vi "Display.vi"() -> ()   [LabVIEW 2009]
panel:
  out "waveform":cluster{i32, dbl, dbl[][]}(graph)
  # "Panel 1"
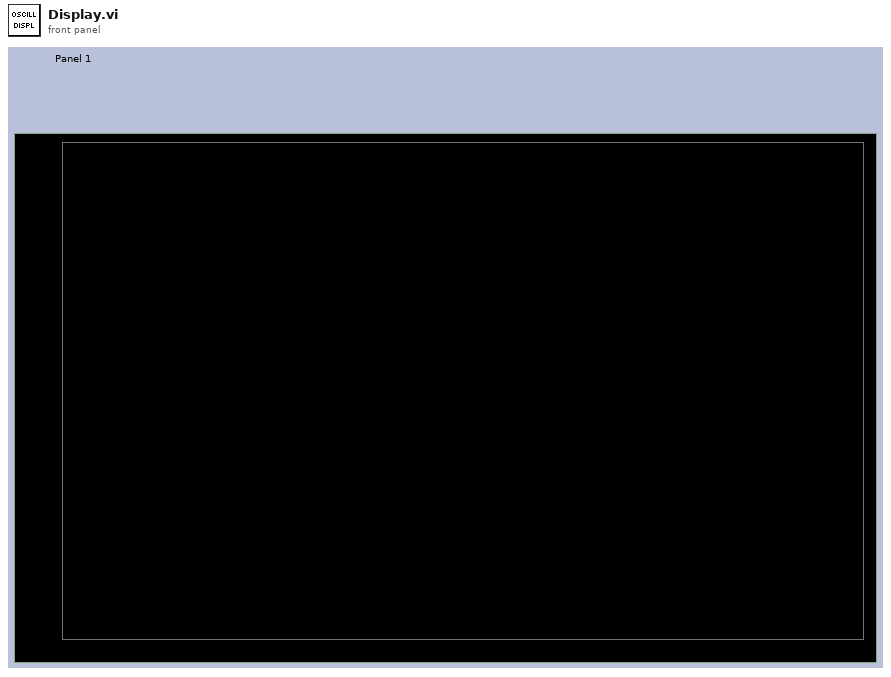
[diagram p1: front panel]
types:
  T1 = cluster{"Minimum":dbl, "Maximum":dbl, "Increment":dbl, "Minor Increment":dbl, "Start":dbl}
  T2 = cluster{"Time Base":u32, "Volts / Div":u32, "Channel In":u32, "Source":bool, "Slope":bool, "Level":dbl}
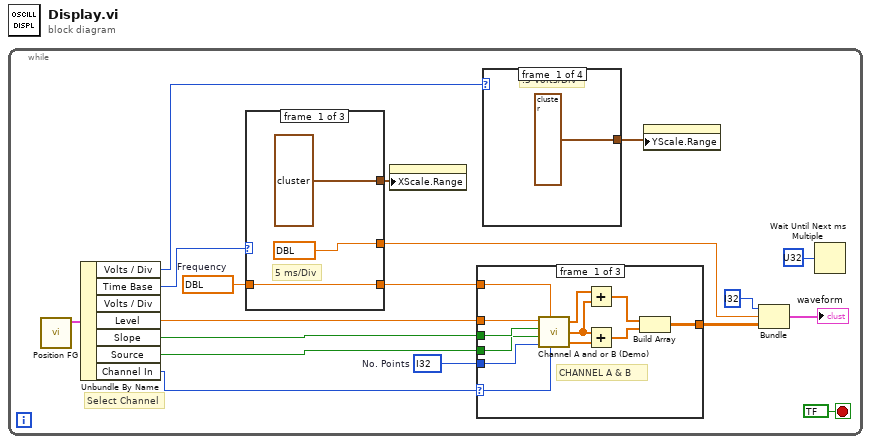
[diagram p0: block diagram]
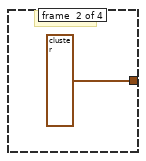
[diagram p2: hidden frame]
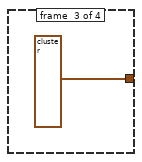
[diagram p3: hidden frame]
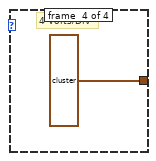
[diagram p4: hidden frame]
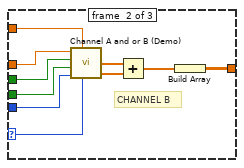
[diagram p5: hidden frame]
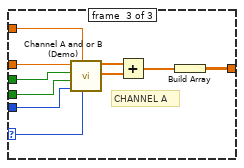
[diagram p6: hidden frame]
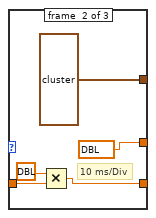
[diagram p7: hidden frame]
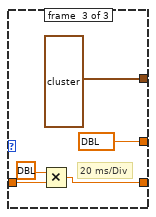
[diagram p8: hidden frame]
diagram:
  n1 = while {
    stop <- bool ? stop-if-true
    w12 = dbl ?  # Frequency
    w18 = i32 ?  # No. Points
    # "Select Channel"
    n2 = call "Position FG.vi"() -> ("Parameters"=w14:T2)  [unwired: 11 in]
    n3 = Unbundle By Name(w14) -> ("Volts / Div"=w2:u32, "Time Base"=w13:u32, "Level"=w3:dbl, "Slope"=w4:bool, "Source"=w5:bool, "Channel In"=w6:u32)  [unwired: 1 out]
    n4 = case shown="2.." w13 {
      tunnel: [w57 w61 w66] -> w17
      tunnel: w12 -> [w57 w62 w67]
      tunnel: [dbl ? dbl ? dbl ?] -> w9
      tunnel: [T1 ? ("Y Scale.Range") T1 ? ("Y Scale.Range") T1 ? ("Y Scale.Range")] -> w15
      frame #0 {
        # "5 ms/Div"
      }
      frame #1 {
        # "10 ms/Div"
        n5 = Multiply(x=dbl ?, y=w62) -> (x*y=w61:dbl)
      }
      frame #2 {
        # "20 ms/Div"
        n6 = Multiply(x=dbl ?, y=w67) -> (x*y=w66:dbl)
      }
    }
    n7 = property on="waveform" class="WFGraph (strict)"("XScale.Range"=w15) -> ()  [unwired: 2 in, 2 out]
    n8 = case shown="2.." w6 {
      selector: w6 -> [w24 w35 w46]
      tunnel: w18 -> [w31 w43 w53]
      tunnel: w17 -> [w23 w36 w45]
      tunnel: w4 -> [w33 w44 w49]
      tunnel: w3 -> [w34 w41 w52]
      tunnel: w5 -> [w32 w42 w54]
      tunnel: [w25 w37 w47] -> w8
      frame #0 {
        # "CHANNEL A & B"
        n9 = call "Channel A and or B (Demo).vi"("Level"=w34, "Frequency"=w23, "Slope"=w33, "Source"=w32, "Select Channel"=w24, "No. Points"=w31) -> ("Waveform 1 Out"=w30:dbl[], "Noise"=w28:dbl[], "Waveform 2 Out"=w29:dbl[])
        n10 = Add(x=w30, y=w28) -> (x+y=w26:dbl[])
        n11 = Add(x=w28, y=w29) -> (x+y=w27:dbl[])
        n12 = Build Array(w26, w27) -> (w25:dbl[][])
      }
      frame #1 {
        # "CHANNEL B"
        n13 = call "Channel A and or B (Demo).vi"("Level"=w41, "Frequency"=w36, "Slope"=w44, "Source"=w42, "Select Channel"=w35, "No. Points"=w43) -> ("Noise"=w40:dbl[], "Waveform 2 Out"=w39:dbl[])  [unwired: 1 out]
        n14 = Add(x=w40, y=w39) -> (x+y=w38:dbl[])
        n15 = Build Array(w38) -> (w37:dbl[][])
      }
      frame #2 {
        # "CHANNEL A"
        n16 = call "Channel A and or B (Demo).vi"("Level"=w52, "Frequency"=w45, "Slope"=w49, "Source"=w54, "Select Channel"=w46, "No. Points"=w53) -> ("Waveform 1 Out"=w51:dbl[], "Noise"=w48:dbl[])  [unwired: 1 out]
        n17 = Add(x=w51, y=w48) -> (x+y=w50:dbl[])
        n18 = Build Array(w50) -> (w47:dbl[][])
      }
    }
    n19 = case shown="2" w2 {
      tunnel: [T1 ? ("Y Scale.Range") T1 ? ("Y Scale.Range") T1 ? ("Y Scale.Range") T1 ? ("Y Scale.Range")] -> w16
      frame #0 {
        # ".5 Volts/Div"
      }
      frame #1 {
        # "1 Volts/Div"
      }
      frame #2 {
      }
      frame #3 {
        # "4 Volts/Div"
      }
    }
    n20 = property on="waveform" class="WFGraph (strict)"("YScale.Range"=w16) -> ()  [unwired: 2 in, 2 out]
    n21 = Bundle(i32 ?, w9, w8) -> (→"waveform":cluster{i32, dbl, dbl[][]})  [unwired: 1 in]
    n22 = Wait Until Next ms Multiple(millisecond multiple=u32 ?) -> ()  [unwired: 1 out]
  }
